vi "OAT Order Magnitude and Phase (Order Waveforms).vi"(0 "order waveforms [EU]":waveform(dbl)[](array[waveform]), 1 "x-axis selection":u16(ring)=2 items=["Time", "Revolution", "RPM"], 5 "speed profile":T12 {"speed [RPM]" format="%.2f"; "time [s]" format="%.2f"}, 7 "pulse/revolution (1)":i32=1, 9 "orders to compute (1.0)":dbl[](array[numeric])=[1.0] format="%.2f", 11 "error in (no error)":errorcluster, 12 "window info":T11={"window type"=62, "window length"=2048} {"window type" items=["None"=0, "Hanning"=1, "Hamming"=2, "Blackman-Harris"=3, "Exact Blackman"=4, "Blackman"=5, "Flat Top"=6, "4 Term B-Harris"=7, "7 Term B-Harris"=8, "Low Sidelobe"=9, "Gaussian"=62]; "window length" min=0}, 13 "view":T10={"dB on? (F)"=FALSE, "unwrap phase? (T)"=TRUE, "unit in degree? (T)"=TRUE}) -> (3 "unit labels":T8, 4 "magnitudes [RMS]":T9(array[cluster]) {"magnitude" format="%.2f"; "time/rev/rpm" format="%.2f"}, 6 "phases [phase lag]":cluster{"time/rev/rpm":dbl[], "phase":dbl[]}[](array[cluster]) {"phase" format="%.2f"; "time/rev/rpm" format="%.2f"}, 8 "magnitude/phase position info":T1, 10 "magnitude info":T2={"channel name"="", "description"="", "x-axis units"=0, "spectral info"={"spectrum type"=enum."Power [Magnitude^2]", "linear/dB"=enum."linear", "window"=0, "window size"=0, "FFT size"=0}, "engineering units"=1, "custom label"="", "dB reference [EU]"=0.0, "peak units"=enum."rms", "weighting filter"=0, "spectral density?"=FALSE, "unit label"="", "spectrum skewed?"=FALSE, "complimentary spectrum units"=enum."none"} {"x-axis units" items=["Time (s)"=0, "Frequency-CB (Hz)"=1, "Frequency-CPB (Hz)"=1248, "Frequency-Arbitrary (Hz)"=2357, "Quefrency (s)"=2, "Revolutions (rev)"=3, "Order"=4, "Speed (RPM)"=11, "Speed (rad/s)"=21, "Index"=65535]; "weighting filter" items=["Linear", "A-weighting", "B-weighting", "C-weighting", "ITU-R 468-4", "Dolby", "CCITT", "C-message", "Wb", "Wc", "Wd", "We", "Wf", "Wh", "Wj", "Wk", "Wm", "AES17 20 kHz lowpass", "AES17 40 kHz lowpass", "AES17 20 kHz highpass", "AES17 40 kHz highpass"]; "dB reference [EU]" format="%.2f"; "engineering units" items=["custom..."=0, "V"=1, "A"=21, "C"=30, "pC"=31, "s"=32, "-"=29, "Pa"=2, "N"=20, "g"=3, "m/s^2"=4, "m/s"=5, "m"=6, "mm/s"=12, "mm"=13, "micron/s"=14, "micron"=15, "in/s^2"=7, "in/s"=8, "in"=9, "mil/s"=10, "mil"=11, "rad/s^2"=16, "rad/s"=17, "rad"=18, "deg/s^2"=26, "deg/s"=27, "deg"=28, "RPM"=22, "cycle/s^2"=23, "Hz"=24, "cycle"=25, "strain"=19]; "spectral info"."window" items=["None "=0, "Hanning"=1, "Hamming"=2, "Blackman-Harris"=3, "Exact Blackman"=4, "Blackman"=5, "Flat Top"=6, "4 Term B-Harris "=7, "7 Term B-Harris"=8, "Low Sidelobe"=9, "Force - Exponential"=10, "Gaussian"=62]}, 15 "error out":errorcluster)   [LabVIEW 2017, in "SoundVib_OrderTracking.lvlib"]
doc: "Computes the magnitudes and phases of designated orders in an even-angle signal. Use this VI to track particular orders specified by <B>orders to compute</B>. Wire data to the <B>even-angle signal</B> input to determine the polymorphic instance to use or manually select the instance."
uses:
  <vilib>/addons/Sound and Vibration/Order Analysis/Resample Order Tracking/SoundVib_OrderTracking.lvlib
  <vilib>/addons/Sound and Vibration/Order Analysis/Tach Process/SubVIs/speed profile.ctl
  <vilib>/addons/Sound and Vibration/Order Analysis/Ref Gabor Order Tracking/window information.ctl
  <vilib>/addons/_NISVFA/_Shared subVIs/Controls/svc_Spectrum Info.ctl
  <vilib>/addons/_NISVFA/_Shared subVIs/Controls/svc_X-Axis Units.ctl
  <vilib>/addons/_NISVFA/_Shared subVIs/Controls/svc_Spectrum Type.ctl
  <vilib>/addons/_NISVFA/_Shared subVIs/Controls/svc_Engineering Units Text Ring.ctl
  <vilib>/addons/_NISVFA/_Shared subVIs/Controls/svc_Weighting Filter Text Ring.ctl
  <vilib>/addons/_NISVFA/_Shared subVIs/Controls/svc_Complimentary Spectrum Units.ctl
  <vilib>/addons/Sound and Vibration/Order Analysis/Misc/OAT Position Info.ctl
  <vilib>/addons/Sound and Vibration/Order Analysis/Resample Order Tracking/SubVIs/OAT Order Magnitude and Phase Plot(XY) (Single Channel).vi
  <vilib>/addons/Sound and Vibration/Order Analysis/Misc/OAT Convert Phase (1 channel).vi
  <vilib>/addons/_NISVFA/_Shared subVIs/Common/svc_Engineering Units to Unit Label.vi
  <vilib>/addons/_NISVFA/_Shared subVIs/Common/svc_Unit Label to Engineering Units.vi
  <vilib>/addons/Sound and Vibration/Order Analysis/Resample Order Tracking/SoundVib_Resampling.lvlib
  <vilib>/addons/Sound and Vibration/Order Analysis/Tach Process/SoundVib_TachProcess.lvlib
  <vilib>/addons/Sound and Vibration/Order Analysis/Gabor Order Tracking/SoundVib_Gabor.lvlib
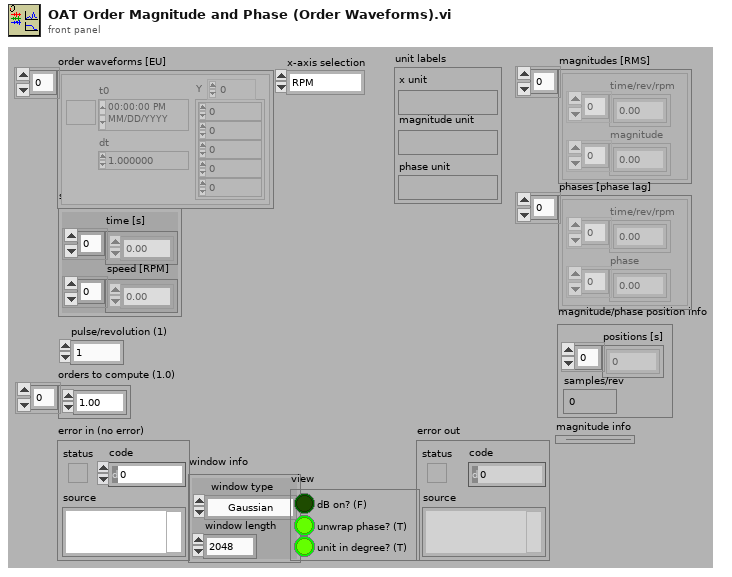
[diagram p1: front panel]
types:
  T1 = typedef "OAT Position Info.ctl" = cluster{"positions [s]":dbl[], "samples/rev":dbl}
  T2 = typedef "svc_Spectrum Info.ctl" = cluster{"channel name":string, "description":string, "x-axis units":T3, "spectral info":cluster{"spectrum type":T4, "linear/dB":enum16{"linear", "dB"}, "window":u16, "window size":i32, "FFT size":i32}, "engineering units":T5, "custom label":string, "dB reference [EU]":dbl, "peak units":enum16{"rms", "peak", "peak-peak"}, "weighting filter":T6, "spectral density?":bool, "unit label":string, "spectrum skewed?":bool, "complimentary spectrum units":T7}
  T3 = typedef "svc_X-Axis Units.ctl" = u16
  T4 = typedef "svc_Spectrum Type.ctl" = enum16{"FFT Spectrum [complex]", "Amplitude [Magnitude]", "Power [Magnitude^2]", "Cross Spectrum [complex]", "Frequency Response [Complex]"}
  T5 = typedef "svc_Engineering Units Text Ring.ctl" = u16
  T6 = typedef "svc_Weighting Filter Text Ring.ctl" = u16
  T7 = typedef "svc_Complimentary Spectrum Units.ctl" = enum16{"none", "radians", "degrees", "cycles", "imaginary"}
  T8 = cluster{"x unit":string, "magnitude unit":string, "phase unit":string}
  T9 = cluster{"time/rev/rpm":dbl[], "magnitude":dbl[]}[]
  T10 = cluster{"dB on? (F)":bool, "unwrap phase? (T)":bool, "unit in degree? (T)":bool}
  T11 = typedef "SoundVib_Gabor.lvlib/window information.ctl" = cluster{"window type":u32, "window length":i32}
  T12 = typedef "SoundVib_TachProcess.lvlib/speed profile.ctl" = cluster{"time [s]":dbl[], "speed [RPM]":dbl[]}
  T13 = cluster{"X unit":string, "unit label":string, string}
  T14 = cluster{"unwrap phase? (T)":bool, "unit in degree? (T)":bool}
  T15 = typedef "svc_Channel Info.ctl" = cluster{"sensor sensitivity":dbl, "engineering units":T5, "dB reference":dbl, "custom label":string, "weighting filter":T6, "pregain":dbl}
  T16 = typedef "svc_Resampled Channel Info.ctl" = cluster{"channel name":string, "description":string, " channel info":T15}
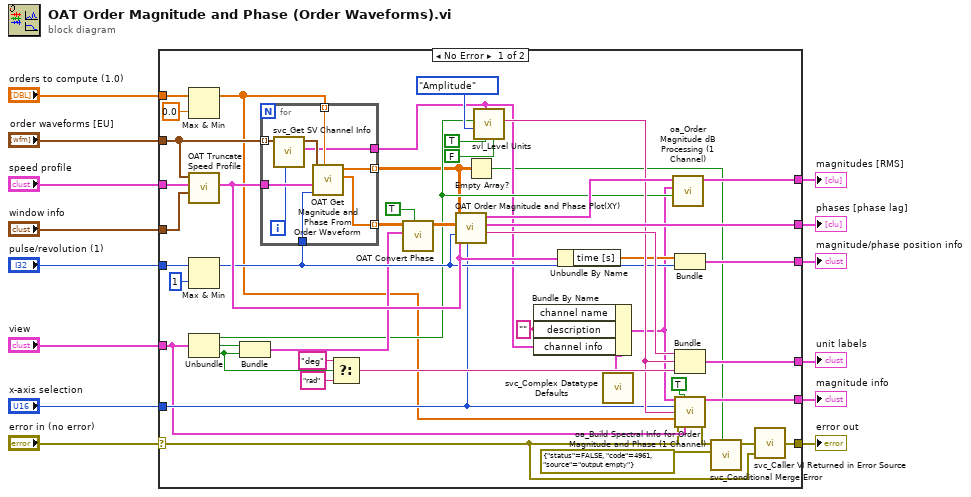
[diagram p0: block diagram]
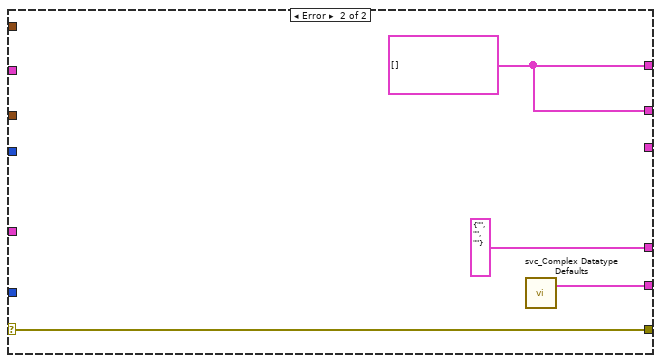
[diagram p2: hidden frame]
diagram:
  n1 = case shown="No Error" "error in (no error)" {
    selector: "error in (no error)" -> [w16 w70]
    tunnel: "window info" -> [w60 _]
    tunnel: "orders to compute (1.0)" -> [w28 _]
    tunnel: "speed profile" -> [w59 _]
    tunnel: [w36 w73] -> w11
    tunnel: [w57 w73] -> w10
    tunnel: "view" -> [w30 _]
    tunnel: "pulse/revolution (1)" -> [w49 _]
    tunnel: [w50 T13 {"X unit"="", "unit label"="", ""}] -> w7
    tunnel: "order waveforms [EU]" -> [w52 _]
    tunnel: [w44 w71] -> w5
    tunnel: [w40 _] -> w4
    tunnel: [w17 w70] -> w3
    tunnel: "x-axis selection" -> [w33 _]
    frame No Error {
      w25 = "" ("channel name")
      n2 = Max & Min(x=w28, y=0.0) -> (max(x,y)=w22:dbl[])  [unwired: 1 out]
      n3 = call <vilib>:"OAT Truncate Speed Profile.vi"("window info"=w60, "speed profile 2"=w59, "order waveforms [EU]"=w52) -> ("speed profile"=w42:T12)  [unwired: 8 in]
      n4 = Max & Min(x=w49, y=1) -> (max(x,y)=w39:i32)  [unwired: 1 out]
      n5 = Unbundle(w30) -> ("dB on? (F)"=w31:bool, "unwrap phase? (T)"=w38:bool, "unit in degree? (T)"=w32:bool)
      n6 = Bundle("unwrap phase? (T)"=w38, "unit in degree? (T)"=w32) -> (w37:T14)  [unwired: 1 in]
      n7 = for {
        tunnel: w39 -> [w66]
        tunnel: w42 -> [w65]
        tunnel: w52 -> [w64] mode=indexing
        tunnel: w22 -> [w69] mode=indexing
        tunnel: [w68] -> w20 mode=indexing
        tunnel: [w67] -> w47 mode=indexing
        tunnel: [w62] -> w24
        i -> [w61]
        n8 = call <vilib>:"svc_Get SV Channel Info.vi"("channel index"=w61, "scaled signal [EU]"=w64) -> ("channel info"=w62:T15, "dup scaled signal [EU]"=w63:waveform(dbl))  [unwired: 4 in, 4 out]
        n9 = call <vilib>:"OAT Get Magnitude and Phase From Order Waveform.vi"("order"=w69, "pulse/revolution (1)"=w66, "speed profile"=w65, "order waveform [EU]"=w63) -> ("phase lag"=w67:dbl[], "magnitudes (RMS)"=w68:dbl[])  [unwired: 6 in]
      }
      n10 = Select(t="deg", s=w32, f="rad") -> (s? t:f=w53:string)
      n11 = call-poly <vilib>:"OAT Convert Phase.vi"("reset (TRUE)"=TRUE, "desired phase setting"=w37, "phase in (rad)"=w47) -> ("phase out"=w46:dbl[][])  [unwired: 8 in]
      n12 = call-poly <vilib>:"OAT Order Magnitude and Phase Plot(XY).vi"("X axis selection"=w33, "speed profile"=w42, "samples/rev"=w39, "phase lag  (even angular)"=w46, "magnitudes (even angular)"=w20) -> ("X unit"=w56:string, "phase lag"=w57:cluster{"X":dbl[], "Y":dbl[]}[], "magnitudes"=w58:cluster{"X":dbl[], "Y":dbl[]}[])  [unwired: 4 in]
      n13 = Empty Array?(array=w20) -> (empty?=w19:bool)
      n14 = call <vilib>:"svl_Level Units.vi"("include weighting if dB On FALSE"=FALSE, "rms level (T)"=TRUE, "channel info"=w24, "view mode"=enum16{"Power", "Amplitude"}."Amplitude", "dB On (T)"=w31) -> ("unit label"=w43:string)  [unwired: 4 in, 2 out]
      n15 = Unbundle By Name(w42) -> ("time [s]"=w41:dbl[])
      n16 = call <vilib>:"svc_Complex Datatype Defaults.vi"() -> ("resampled channel info"=w26:T16)  [unwired: 11 in, 8 out]
      n17 = Bundle By Name(cluster=w26, "channel name"=w25, "description"=w25, "channel info"=w24) -> (w23:T16)
      n18 = call <vilib>:"oa_Order Magnitude dB Processing (1 Channel).vi"("dB on? (T)"=w31, "even angle channel info"=w23, "magnitudes"=w58) -> ("magnitudes dB"=w36:T9)  [unwired: 8 in]
      n19 = Bundle("time [s]"=w41, w39) -> (w40:cluster{"time [s]":dbl[], i32})  [unwired: 1 in]
      n20 = Bundle("X unit"=w56, "unit label"=w43, w53) -> (w50:T13)  [unwired: 1 in]
      n21 = call <vilib>:"oa_Build Spectral Info for Order Magnitude and Phase (1 Channel).vi"("resampled channel info"=w23, "reset? (T)"=TRUE, "X axis selection"=w33, "unit label"=w43, "orders to compute"=w22, "error in (no error)"=w16, "view"=w30) -> ("spectrum info"=w44:T2, "error out"=w21:errorcluster)  [unwired: 7 in]
      n22 = call <vilib>:"svc_Conditional Merge Error.vi"("merge"=w19, "new error"=errorcluster {"status"=FALSE, "code"=4961, "source"="output empty"}, "error in (no error)"=w21) -> ("error out"=w18:errorcluster)  [unwired: 8 in]
      n23 = call <vilib>:"svc_Caller VI Returned in Error Source.vi"("warning input to caller"=w16, "error in (no error)"=w18) -> ("error out"=w17:errorcluster)  [unwired: 3 in]
    }
    frame Error {
      w73 = cluster{"X":dbl[], "Y":dbl[]}[] [] ("magnitudes")
      n24 = call <vilib>:"svc_Complex Datatype Defaults.vi"() -> ("dead spectrum info"=w71:T2)  [unwired: 11 in, 8 out]
    }
  }
  "magnitudes [RMS]" <- w11
  "phases [phase lag]" <- w10
  "unit labels" <- w7
  "error out" <- w3
  "magnitude info" <- w5
  "magnitude/phase position info" <- w4
